vi "Create JV folder.vi"(11 "Data Folder In":path) -> (3 "Data Output Folder":path)   [LabVIEW 2011]
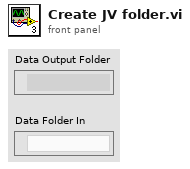
[diagram p1: front panel]
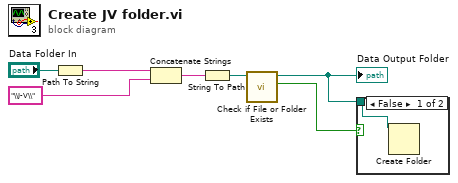
[diagram p0: block diagram]
diagram:
  n1 = Path To String(path="Data Folder In") -> (string=w2:string)
  n2 = Concatenate Strings(w2, "\\J-V\\") -> (w5:string)
  n3 = String To Path(string=w5) -> (path=w6:path)
  n4 = call <vilib>:"Check if File or Folder Exists.vi"("path"=w6) -> ("file or folder exists?"=w7:bool, "dup path"=w4:path)  [unwired: 8 in, 1 out]
  "Data Output Folder" <- w4
  n5 = case shown="False" w7 {
    tunnel: w4 -> [w8 _]
    frame False {
      n6 = Create Folder(path (use dialog)=w8) -> ()  [unwired: 2 in, 3 out]
    }
    frame True {
    }
  }
